vi "ProgG_008_MG.vi"() -> ()   [LabVIEW 2021]
panel:
  out "Czas obliczeń [s]":dbl=0.101
  in  "Różnica ciągu arytmetycznego":dbl=6.0
  in  "Pierwszy wyraz":dbl=5.0
  in  "Któy wyraz ciągu obliczyć?\nN":i64=99999999
  out "Obliczony wyraz ciągu":i64=599999993
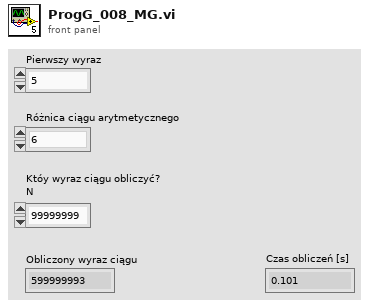
[diagram p1: front panel]
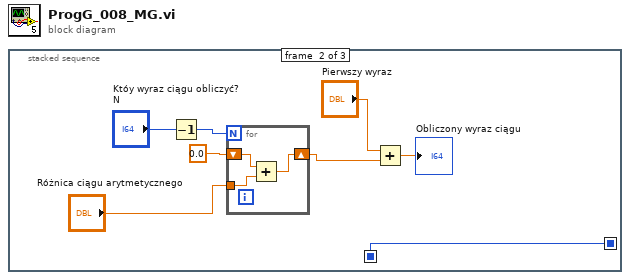
[diagram p0: block diagram]
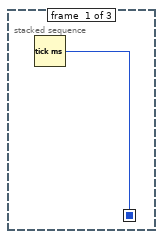
[diagram p2: hidden frame]
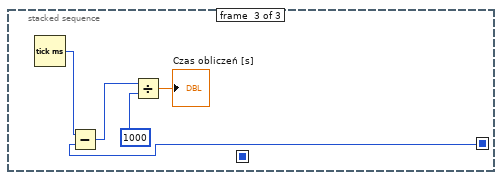
[diagram p3: hidden frame]
diagram:
  n1 = stacked-sequence {
    seq-local: [w1 _ _] -> [_ w9 _]
    seq-local: [_ w9 _] -> [_ _ w17]
    frame #0 {
      n2 = Tick Count (ms)() -> (millisecond timer value=w1:u32)
    }
    frame #1 {
      n3 = Decrement(x="Któy wyraz ciągu obliczyć?\nN") -> (x-1=w5:i64)
      n4 = for {
        N: w5 -> [_]
        tunnel: "Różnica ciągu arytmetycznego" -> [w12]
        shift-right: [w10] -> w2
        shift-left: 0.0 ("x") -> [w11]
        n5 = Add(x=w11, y=w12) -> (x+y=w10:dbl)
      }
      n6 = Add(x="Pierwszy wyraz", y=w2) -> (x+y=→"Obliczony wyraz ciągu":dbl)
    }
    frame #2 {
      n7 = Tick Count (ms)() -> (millisecond timer value=w16:u32)
      n8 = Subtract(x=w16, y=w17) -> (x-y=w14:u32)
      n9 = Divide(x=w14, y=u32 1000) -> (x/y=→"Czas obliczeń [s]":dbl)
    }
  }
